vi "Configure Trigger.vi"(0 "VISA resource name":refnum<visa-resource-name>, 1 "Trigger Source (0: Immediate)":u16(ring) items=["Immediate", "Manual", "External", "Bus", "LEVEL", "DELTA"], 3 "Sample Count (1)":u32=1 min=1 max=16000 step=1, 4 "Disable Trig Delay (T: Disable)":bool=TRUE, 5 "error in (no error)":errorcluster, 7 "Trigger Delay (0.0 s)":dbl min=0.0 max=3600.0 step=1e-05 format="%_6g", 8 "Pre Trigger (0: 0%)":u16(ring) items=["0% (OFF)", "25%", "50%", "75%"], 9 "DELTA Trigger Pattern (1: Emission )":u16(ring)=1 items=["CONVERGE", "EMISSION"], 10 "Level Count (0)":i32 min=-319999 max=319999, 11 "Delta Count (1)":i32=1 min=1 max=160000, 12 "LEVL Trigger Slope (1: Positive )":u16(ring)=1 items=[" NEGATIVE (Falling slope)", "POSITIVE (Rising slope)"], 13 "DELTA Trigger Slope (1: Positive )":u16(ring)=1 items=["NEGATIVE (Falling slope)", "POSITIVE (Rising slope)", "BOTH (absolute value)"]) -> (14 "VISA resource name out":refnum<visa-resource-name>, 19 "error out":errorcluster)   [LabVIEW 2017, in "ADCMT7451_ADC.lvlib"]
doc: "Configures the trigger settings on the instrument.\n\n<B>Note:</B> Use this VI only with other low-level VIs. The high-level VIs automatically incorporate this functionality."
uses:
  ADCMT7451_ADC.lvlib
panel:
  in  "Parameters for LEVEL/DELTA Trigger":enum32{"for LEVEL", "for DELTA"}(tab)
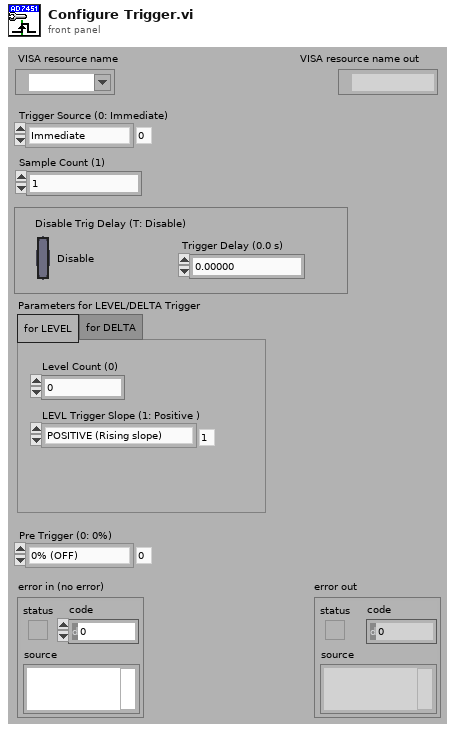
[diagram p1: front panel]
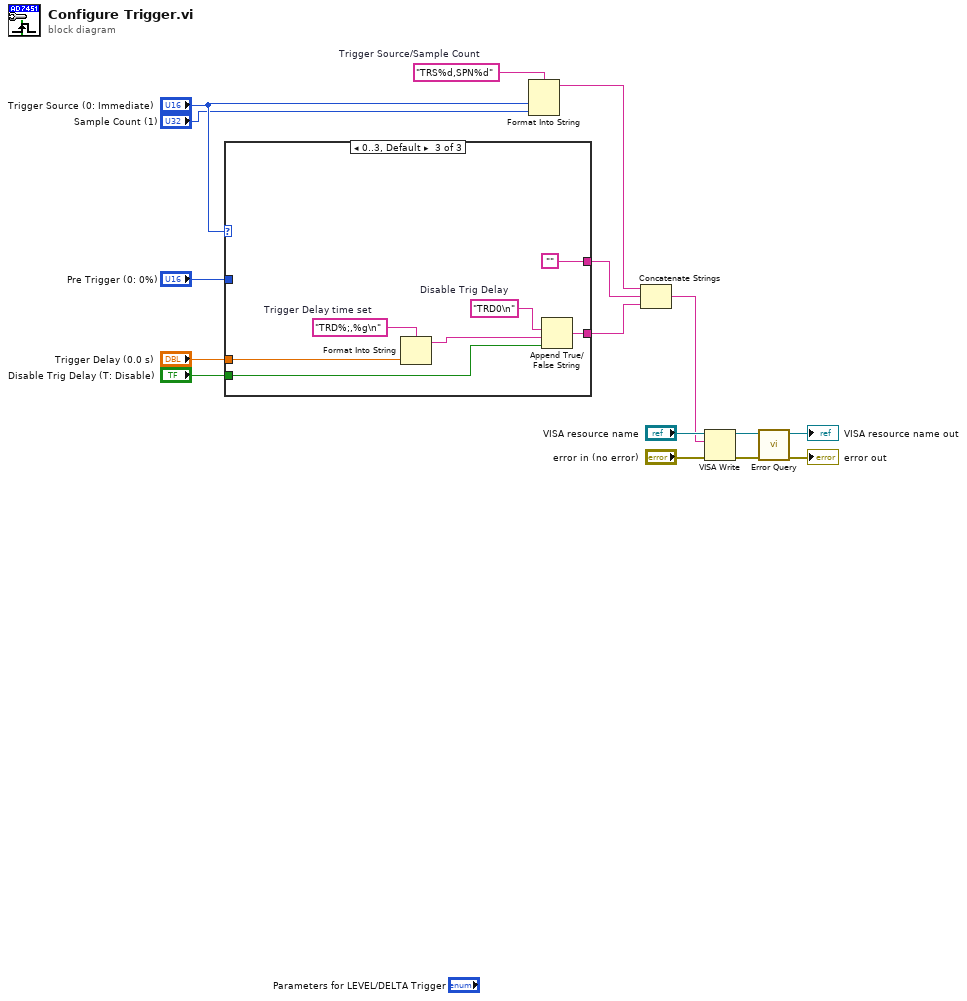
[diagram p0: block diagram]
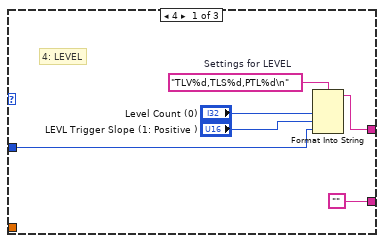
[diagram p2: hidden frame]
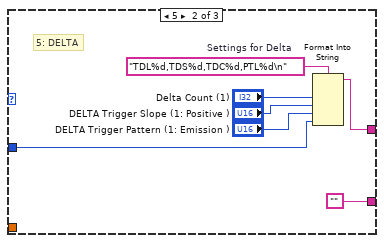
[diagram p3: hidden frame]
diagram:
  w10 = "TRS%d,SPN%d"  # Trigger Source/Sample Count
  n1 = case shown="0..3, Default" "Trigger Source (0: Immediate)" {
    tunnel: [w17 w23 ""] -> w8
    tunnel: "Pre Trigger (0: 0%)" -> [w19 w26 _]
    tunnel: ["" "" w32] -> w5
    tunnel: "Disable Trig Delay (T: Disable)" -> [_ _ w31]
    tunnel: "Trigger Delay (0.0 s)" -> [_ _ w30]
    frame 4 {
      w22 = "TLV%d,TLS%d,PTL%d\n"  # Settings for LEVEL
      # "4: LEVEL"
      n2 = Format Into String(format string=w22, "Level Count (0)", "LEVL Trigger Slope (1: Positive )", w19) -> (resulting string=w17:string)  [unwired: 2 in, 1 out]
    }
    frame 5 {
      w29 = "TDL%d,TDS%d,TDC%d,PTL%d\n"  # Settings for Delta
      # "5: DELTA"
      n3 = Format Into String(format string=w29, "Delta Count (1)", "DELTA Trigger Slope (1: Positive )", "DELTA Trigger Pattern (1: Emission )", w26) -> (resulting string=w23:string)  [unwired: 2 in, 1 out]
    }
    frame 0..3, Default {
      w34 = "TRD0\n"  # Disable Trig Delay
      w33 = "TRD%;,%g\n"  # Trigger Delay time set
      n4 = Format Into String(format string=w33, w30) -> (resulting string=w35:string)  [unwired: 2 in, 1 out]
      n5 = Append True/False String(1:w31, 2:w35, 3:w34) -> (0:w32:string)  [unwired: 1 in]
    }
  }
  n6 = Format Into String(format string=w10, "Trigger Source (0: Immediate)", "Sample Count (1)") -> (resulting string=w2:string)  [unwired: 2 in, 1 out]
  n7 = Concatenate Strings(w2, w8, w5) -> (w7:string)
  n8 = VISA Write(VISA resource name="VISA resource name", write buffer=w7, error in (no error)="error in (no error)") -> (VISA resource name out=w12:refnum<visa-resource-name>, error out=w11:errorcluster)  [unwired: 1 out]
  n9 = call "Error Query.vi"("error in (no error)"=w11, "VISA resource name"=w12) -> ("error out"=→"error out":errorcluster, "VISA resource name out"=→"VISA resource name out":refnum<visa-resource-name>)  [unwired: 6 in, 2 out]
